vi "2D Error Bar Plot.vi"() -> ()   [LabVIEW 2017, in "2D_Merge.lvlib"]
uses:
  <vilib>/Math Plots/2D Math Plots/Merge VIs/2D_Merge.lvlib
  <vilib>/Math Plots/2D Math Plots/2D Error Bar/2D Error Bar XCtrl/2D Error Bar.xctl
  <vilib>/Math Plots/2D Math Plots/2D Error Bar/2D Error Bar Datatype/Public/Plot Helper (Percentage).vi
  <vilib>/Math Plots/2D Math Plots/2D Error Bar/2D Error Bar Datatype/2D Error Bar Datatype.lvclass
panel:
  out "2D Error Bar":refnum<class "2D Plot Datatype.lvclass">[](xcontrol)
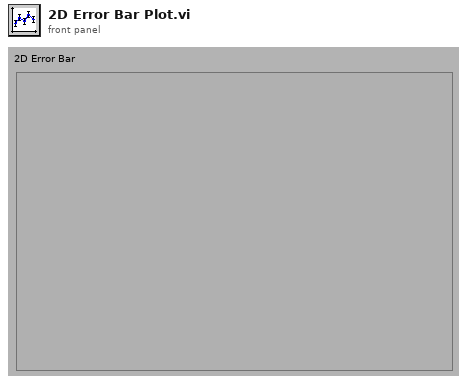
[diagram p1: front panel]
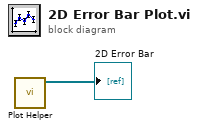
[diagram p0: block diagram]
diagram:
  n1 = call-poly <vilib>:"Plot Helper.vi"() -> ("2D Plot Class Obj Array out"=→"2D Error Bar":refnum<class "2D Plot Datatype.lvclass">[])  [unwired: 6 in, 5 out]
